vi "Build Line.vi"(6 "Value String (\"\")":string, 8 "Name In":string, 9 "Array":u32[](array[numeric]), 10 "Iteration":i32, 11 "Iterations":i32) -> (0 "Line":string, 1 "Name Out":string)   [LabVIEW 2009]
doc: "This VI was created for use with the Read/Write Cluster VIs. It builds the key name and value line for the INI file for arrays.\n\nFreeware from Moore Good Ideas, www.mooregoodideas.com. Do not remove this line."
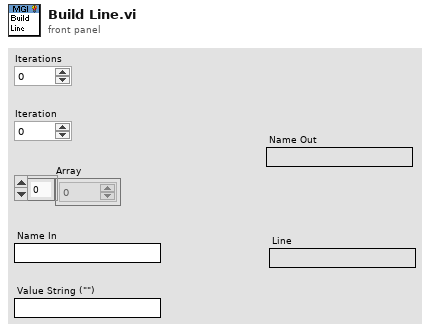
[diagram p1: front panel]
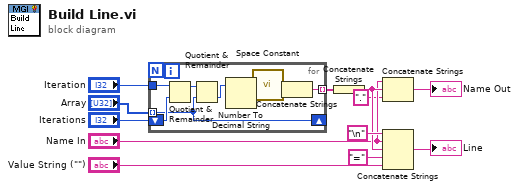
[diagram p0: block diagram]
diagram:
  n1 = for {
    tunnel: [w19] -> w9 mode=indexing
    tunnel: "Iteration" -> [w16]
    tunnel: "Array" -> [w13] mode=indexing
    shift-right: [w13] -> _
    shift-left: "Iterations" -> [w15]
    n2 = Quotient & Remainder(x=w16, y=w15) -> (x-y*floor(x/y)=w17:u32)  [unwired: 1 out]
    n3 = Quotient & Remainder(x=w17, y=w13) -> (floor(x/y)=w14:u32)  [unwired: 1 out]
    n4 = Number To Decimal String(number=w14) -> (decimal integer string=w20:string)  [unwired: 1 in]
    n5 = call <vilib>:"Space Constant.vi"() -> ("String"=w18:string)
    n6 = Concatenate Strings(w18, w20) -> (w19:string)
  }
  n7 = Concatenate Strings(w9) -> (w3:string)
  n8 = Concatenate Strings("Name In", w3, "." ("string")) -> (→"Name Out":string)
  n9 = Concatenate Strings("\n", "Name In", w3, "=" ("string"), "Value String (\"\")") -> (→"Line":string)
